vi "Close.vi"(8 "error in":errorcluster, 11 "Measure":refnum<class "Measure.lvclass">) -> (0 "error out":errorcluster)   [LabVIEW 2021, in "ProligentXMLGenerator.lvlib" / "Measure.lvclass"]
uses:
  Measure.lvclass
  Measure.lvclass/Measure.ctl
  Model/Characteristic/Characteristic.lvclass
  Failure/FailureReference/FailureReference.lvclass
  Model/CustomData/CustomData.lvclass
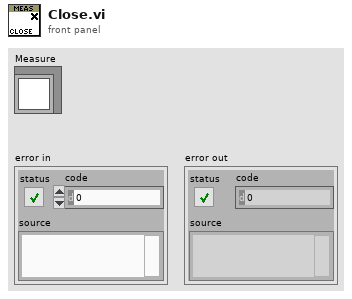
[diagram p1: front panel]
types:
  T1 = typedef "ProligentXMLGenerator.lvlib/Measure.lvclass/Data.ctl" = cluster{"Name":string, "Type":refnum<class "MeasureKind.lvclass">, "Precision":refnum<class "UnsignedByte.lvclass">, "Limit":refnum<class "MeasureLimit.lvclass">, "Characteristics":refnum<class "Characteristic.lvclass">[], "FailureReferences":refnum<class "FailureReference.lvclass">[], "CustomData":refnum<class "CustomData.lvclass">, "MeasureId":refnum<class "Guid.lvclass">, "MeasureTime":refnum<class "DateTime.lvclass">, "Comments":refnum<class "NonNullableString_TruncateAt_255.lvclass">, "Unit":refnum<class "NonEmptyString_30.lvclass">, "Symbol":refnum<class "NonEmptyString_20.lvclass">, "MeasureExecutionStatus":refnum<class "ExecutionStatus.lvclass">}
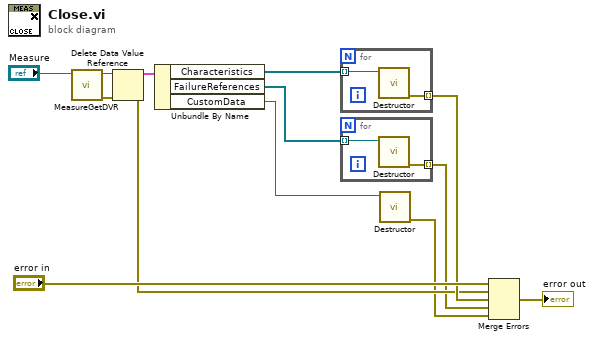
[diagram p0: block diagram]
diagram:
  n1 = call "MeasureGetDVR.vi"("Measure"="Measure") -> ("error out"=w10:errorcluster, "DVRReference"=w11:refnum<data-value>)  [unwired: 9 in]
  n2 = Delete Data Value Reference(data value reference=w11, error in=w10) -> (data value=w8:T1, error out=w6:errorcluster)
  n3 = Unbundle By Name(w8) -> ("Characteristics"=w5:refnum<class "Characteristic.lvclass">[], "FailureReferences"=w4:refnum<class "FailureReference.lvclass">[], "CustomData"=w1:refnum<class "CustomData.lvclass">)
  n4 = for {
    tunnel: w5 -> [w15] mode=indexing
    tunnel: [w14] -> w7 mode=indexing
    n5 = call "Destructor.vi"("Document in"=w15) -> ("error out"=w14:errorcluster)  [unwired: 10 in]
  }
  n6 = for {
    tunnel: w4 -> [w17] mode=indexing
    tunnel: [w16] -> w3 mode=indexing
    n7 = call "Destructor.vi"("FailureReference in"=w17) -> ("error out"=w16:errorcluster)  [unwired: 10 in]
  }
  n8 = call "Destructor.vi"("CustomDataType"=w1) -> ("error out"=w2:errorcluster)  [unwired: 10 in]
  n9 = Merge Errors("error in", w6, w7, w3, w2) -> (→"error out":errorcluster)
